vi "SR400 Control.vi"(0 "VISA Port In":refnum<visa-resource-name>="GPIB0::23::INSTR", 11 "error in":errorcluster) -> (4 "VISA Port Out":refnum<visa-resource-name>="SR400", 15 "error out":errorcluster)   [LabVIEW 2019]
doc: "Ce VI sert de centrale de contrôle pour le compteur de photon SR400. Il permet à l'usager de régler les différnet paramètres de comptage, de porte et de discriminateur."
uses:
  <vilib>/Utility/error.llb/DialogType.ctl
panel:
  in  "ReadPar":bool
  in  "Test":bool
  in  "BGatePar":T1={"Mode"=0, "Durée"=0.9992, "Délais"=0.9992, "Incrément"=0.9992} caption="Paramètres de la porte d'acquisition «B»" {"Incrément" min=0.0 max=0.9992 step=1e-09 format="%#_4g"; "Délais" min=0.0 max=0.9992 step=1e-09 format="%#_4g"; "Durée" min=5e-09 max=0.9992 step=1e-09 format="%#_4g"; "Mode" items=["CW", "Fixed", "Scan"]}
  in  "AGatePar":T1={"Mode"=0, "Durée"=0.9992, "Délais"=0.9992, "Incrément"=0.9992} caption="Paramètres de la porte d'acquisition «A»" {"Incrément" min=0.0 max=0.9992 step=1e-09 format="%#_4g"; "Délais" min=0.0 max=0.9992 step=1e-09 format="%#_4g"; "Durée" min=5e-09 max=0.9992 step=1e-09 format="%#_4g"; "Mode" items=["CW", "Fixed", "Scan"]}
  in  "Discriminateur T":T2 {"Incrément (V)" min=-0.02 max=0.02 step=0.0002; "Niveau (V)" min=-0.3 max=0.3 step=0.0002; "Front A" items=["Montant", "Descendant"]; "Mode" items=["Fixe", "Scan"]}
  in  "Discriminateur B":T2 {"Incrément (V)" min=-0.02 max=0.02 step=0.0002; "Niveau (V)" min=-0.3 max=0.3 step=0.0002; "Front A" items=["Montant", "Descendant"]; "Mode" items=["Fixe", "Scan"]}
  in  "Discriminateur A":T2 {"Incrément (V)" min=-0.02 max=0.02 step=0.0002; "Niveau (V)" min=-0.3 max=0.3 step=0.0002; "Front A" items=["Montant", "Descendant"]; "Mode" items=["Fixe", "Scan"]}
  in  "Counter T Preset (s)":dbl=0.001 min=1e-07 max=90000.0 step=1e-07 format="%#.7g"
  in  "Dwell time":dbl=6.0 caption="\"Dwell Time\" (s)" min=0.002 max=6.0 step=0.001
  in  "Mode":u16(ring) items=["A,B for T Preset", "A-B for T Preset", "A+B for T Preset", "A for B preset"]
  in  "Nb de période":i32=1 min=1 max=2000 step=1
  in  "Counter B Preset (s)":dbl=0.001 min=1e-07 max=90000.0 step=1e-07 format="%#.7g"
  in  "T Source":u16(ring) caption="Source «T»" items=["10 MHz"=0, "Input 2"=2, "Trig"=3]
  in  "B Source":u16(ring)=2 caption="Source «B»" items=["Input 1"=1, "Input 2"=2]
  in  "A Source":u16(ring)=1 caption="Source «A»" items=["Input 1"=1, "10 MHz"=0]
  in  "Quit":bool
  # "Panneaux de contrôle du Compteur de Photon SR400"
  # "Porte D'acquisition «Gate»"
  # "Source de comptage"
  # "Paramètres de comptage"
  # "Discriminateur"
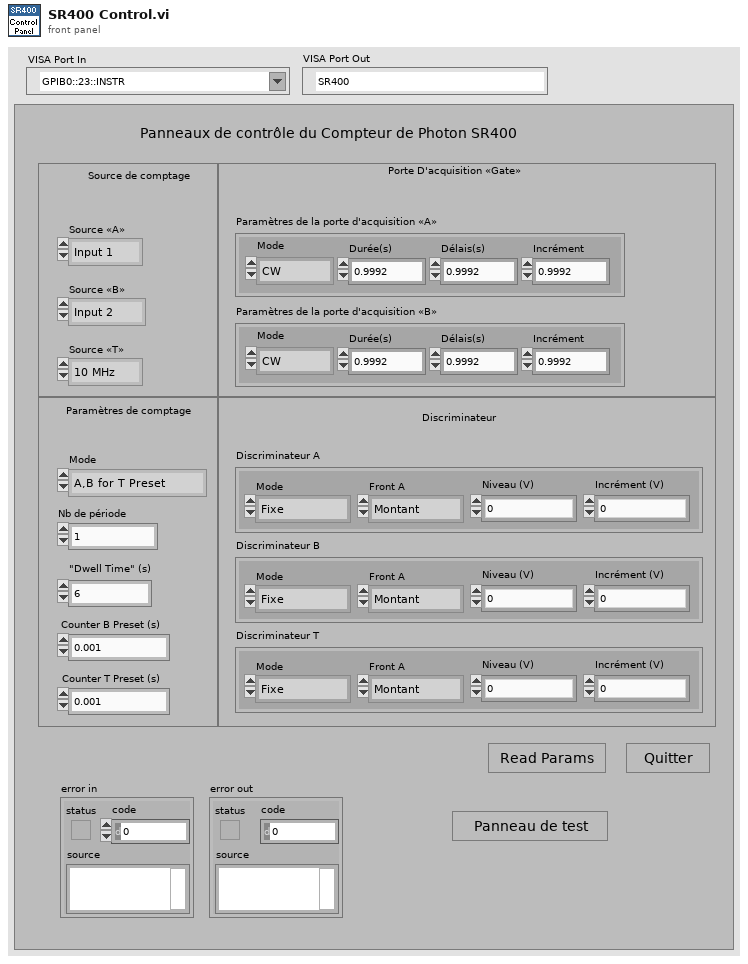
[diagram p1: front panel]
types:
  T1 = cluster{"Mode":u16, "Durée":dbl, "Délais":dbl, "Incrément":dbl}
  T2 = cluster{"Mode":u16, "Front A":u16, "Niveau (V)":dbl, "Incrément (V)":dbl}
  T3 = enum16{"All", "Mode", "T Preset", "B Preset", "Dwell", "NbPeriod", "Counter"}
  T4 = typedef "DialogType.ctl" = u16
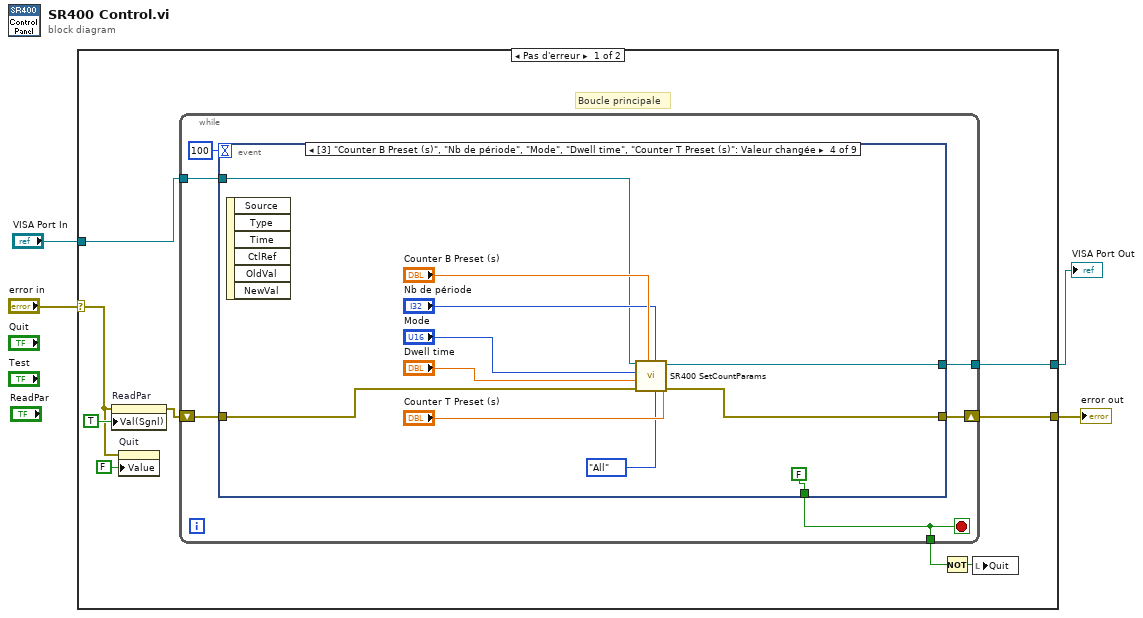
[diagram p0: block diagram]
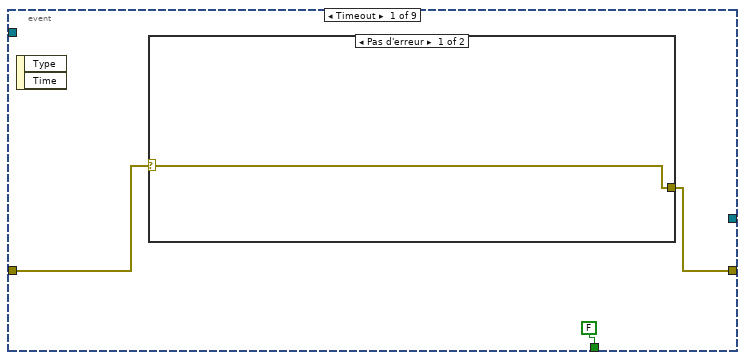
[diagram p2: hidden frame]
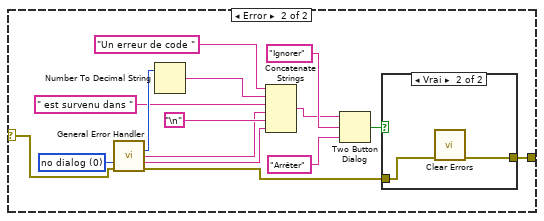
[diagram p3: hidden frame]
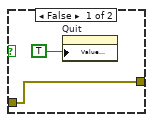
[diagram p4: hidden frame]
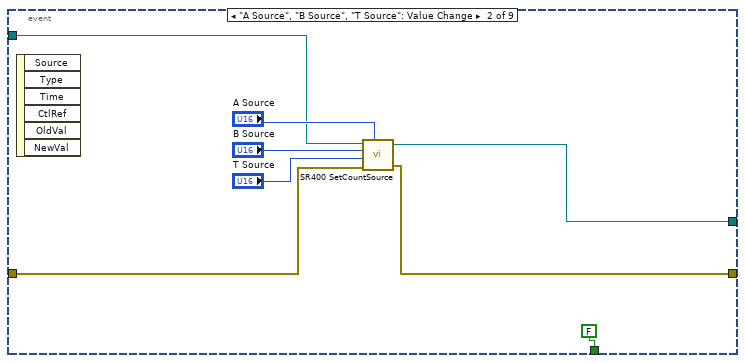
[diagram p5: hidden frame]
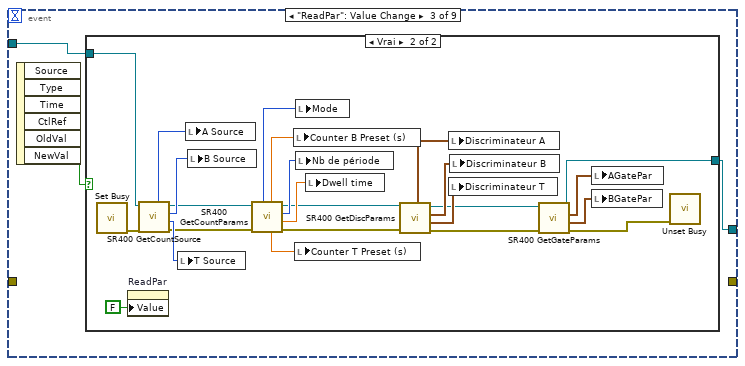
[diagram p6: hidden frame]
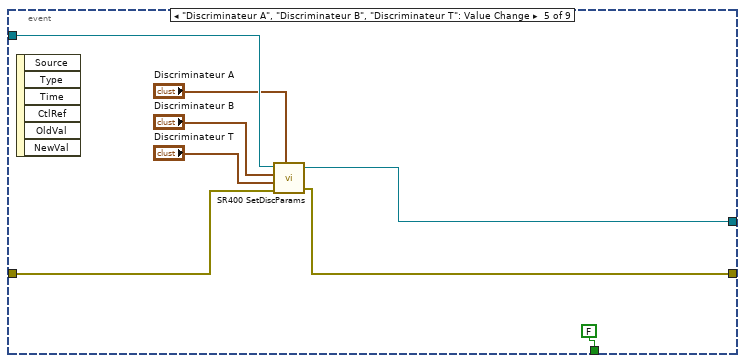
[diagram p8: hidden frame]
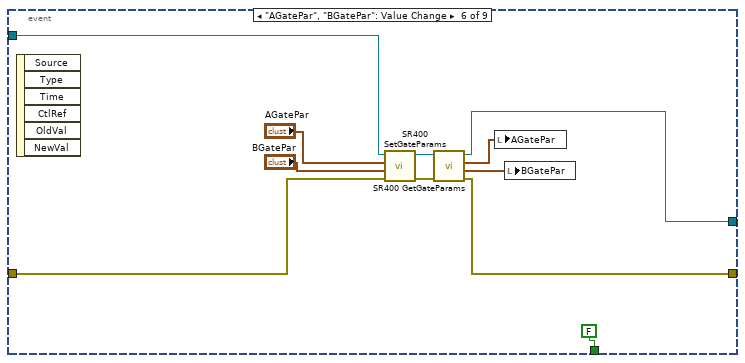
[diagram p9: hidden frame]
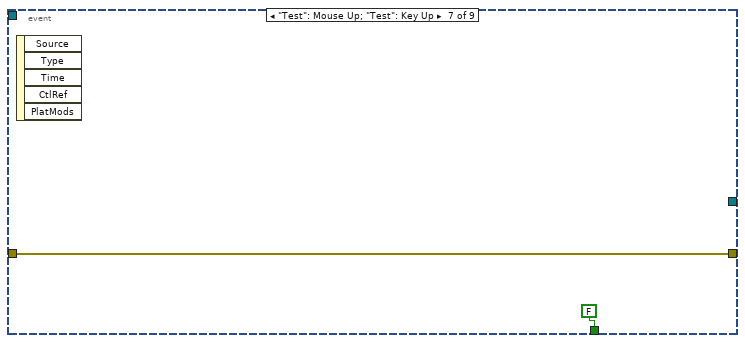
[diagram p10: hidden frame]
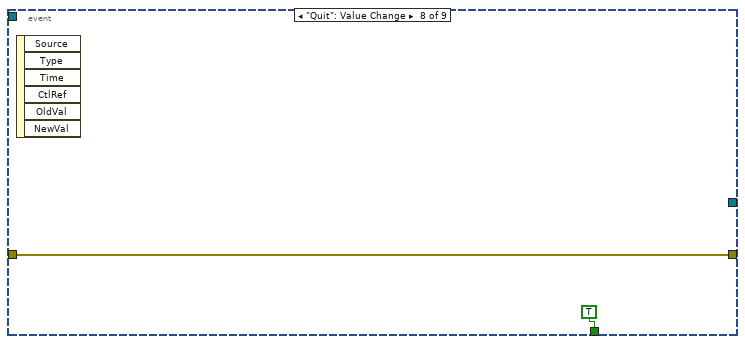
[diagram p11: hidden frame]
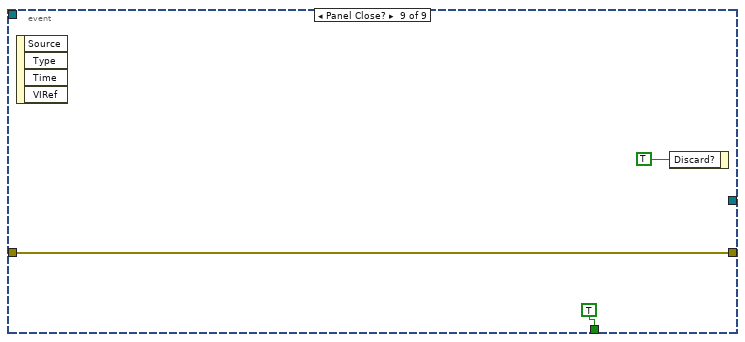
[diagram p12: hidden frame]
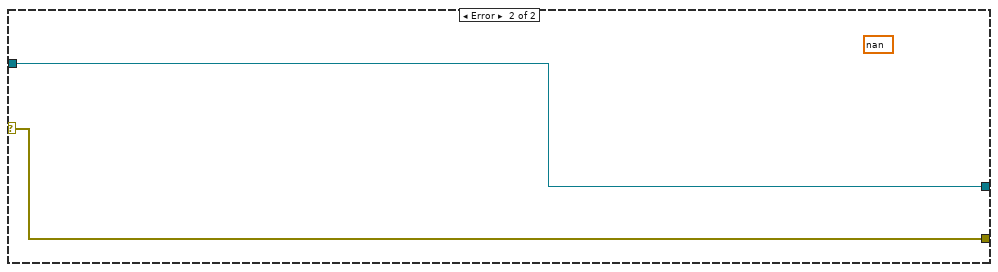
[diagram p13: hidden frame]
diagram:
  n1 = case shown="Pas d'erreur" "error in" {
    selector: "error in" -> [w5 w117]
    tunnel: [w13 w117] -> w3
    tunnel: "VISA Port In" -> [w7 w116]
    tunnel: [w12 w116] -> w1
    frame No Error {
      # "Boucle principale"
      n2 = property on="ReadPar" class="Bool (strict)"(error in=w5, "Val(Sgnl)"=TRUE ("Value (Signaling)")) -> (error out=w9:errorcluster)  [unwired: 1 in, 1 out]
      n3 = property on="Quit" class="Bool (strict)"(error in=w5, "Value"=FALSE ("Quit")) -> ()  [unwired: 1 in, 2 out]
      n4 = while {
        shift-right: [w17] -> w13
        shift-left: w9 -> [w18]
        tunnel: [w16] -> w11
        tunnel: w7 -> [w15]
        tunnel: [w14] -> w12
        stop <- w16 stop-if-true
        n5 = event shown="[3] \"Counter B Preset (s)\", \"Nb de période\", \"Mode\", \"Dwell time\", \"Counter T Preset (s)\": Valeur changée" {
          selector: _ -> [_ _ _ _ _ _ _ _ _]
          dyn-events: _ -> [_ _ _ _ _ _ _ _ _]
          timeout: 100 -> [_ _ _ _ _ _ _ _ _]
          tunnel: w18 -> [w20 w50 _ w89 w97 w108 w109 w111 w113]
          tunnel: [w21 w49 _ w88 w96 w106 w109 w111 w113] -> w17
          tunnel: [FALSE ("status") FALSE ("status") _ FALSE ("status") FALSE ("status") FALSE ("status") FALSE ("status") TRUE ("status") TRUE ("status")] -> w16
          tunnel: w15 -> [_ w44 w53 w81 w92 w101 _ _ _]
          tunnel: [_ w43 w52 w80 w90 w103 _ _ _] -> w14
          event Timeout {
            n6 = event-data() -> ()  [unwired: 1 in, 2 out]
            n7 = case shown="Pas d'erreur" w20 {
              selector: w20 -> [w23 w24]
              tunnel: [w23 w25] -> w21
              frame No Error {
              }
              frame Error {
                w35 = T4 0 items=["no dialog", "OK message", "continue or stop message", "OK message + warnings", "continue/stop + warnings"] ("type of dialog (OK msg:1)")
                n8 = call <vilib>:"General Error Handler.vi"("type of dialog (OK msg:1)"=w35, "error in (no error)"=w24) -> ("code out"=w31:i32, "source out"=w30:string, "message"=w28:string, "error out"=w26:errorcluster)  [unwired: 9 in, 1 out]
                n9 = Number To Decimal String(number=w31) -> (decimal integer string=w32:string)  [unwired: 1 in]
                n10 = Concatenate Strings("Un erreur de code " ("string"), w32, " est survenu dans " ("string"), w30, "\n", w28) -> (w27:string)
                n11 = Two Button Dialog(message=w27, 1:"Arrêter" ("F button name (\"Cancel\")"), 2:"Ignorer" ("T button name (\"OK\")")) -> (T button?=w38:bool)
                n12 = case shown="Vrai" w38 {
                  tunnel: w26 -> [w40 w42]
                  tunnel: [w40 w41] -> w25
                  frame False {
                    n13 = property on="Quit" class="Bool (strict)"("Value (Signaling)"=TRUE) -> ()  [unwired: 2 in, 2 out]
                  }
                  frame True {
                    n14 = call <vilib>:"Clear Errors.vi"("error in (no error)"=w42) -> ("error out"=w41:errorcluster)  [unwired: 5 in, 1 out]
                  }
                }
              }
            }
          }
          event "A Source", "B Source", "T Source": Value Change {
            n15 = event-data() -> ()  [unwired: 1 in, 6 out]
            n16 = call <userlib>:"SR400 SetCountSource.vi"("error in (no error)"=w50, "T Source"="T Source", "A Source"="A Source", "B Source"="B Source", "VISA Port In"=w44) -> ("error out"=w49:errorcluster, "VISA Port Out"=w43:refnum<visa-resource-name>)  [unwired: 4 in]
          }
          event "ReadPar": Value Change {
            n17 = event-data() -> ("NewVal"=w51:bool)  [unwired: 1 in, 5 out]
            n18 = case shown="Vrai" w51 {
              tunnel: w53 -> [w54 w58]
              tunnel: [w54 w57] -> w52
              frame False {
              }
              frame True {
                n19 = call <vilib>:"Set Busy.vi"() -> ("error out"=w69:errorcluster)  [unwired: 10 in, 1 out]
                n20 = property on="ReadPar" class="Bool (strict)"("Value"=FALSE ("ReadPar")) -> ()  [unwired: 2 in, 2 out]
                n21 = call <userlib>:"SR400 GetCountSource.vi"("error in (no error)"=w69, "VISA Port In"=w58) -> ("error out"=w77:errorcluster, "T Source"=w78:u16, "B Source"=w67:u16, "VISA Port Out"=w66:refnum<visa-resource-name>, "A Source"=w68:u16)  [unwired: 4 in]
                n22 = local write "T Source"(w78) -> ()
                n23 = local write "A Source"(w68) -> ()
                n24 = local write "B Source"(w67) -> ()
                n25 = call <userlib>:"SR400 GetCountParams.vi"("error in (no error)"=w77, "VISA Port In"=w66) -> ("error out"=w74:errorcluster, "Dwell time"=w76:dbl, "Nb de période"=w75:i32, "VISA Port Out"=w62:refnum<visa-resource-name>, "CounterPresT"=w64:dbl, "CounterPresB"=w65:dbl, "Mode"=w63:u16)  [unwired: 3 in]
                n26 = local write "Counter B Preset (s)"(w65) -> ()
                n27 = local write "Counter T Preset (s)"(w64) -> ()
                n28 = local write "Mode"(w63) -> ()
                n29 = local write "Nb de période"(w75) -> ()
                n30 = local write "Dwell time"(w76) -> ()
                n31 = call <userlib>:"SR400 GetDiscParams.vi"("error in (no error)"=w74, "VISA Port In"=w62) -> ("error out"=w70:errorcluster, "Discriminateur T"=w71:T2, "Discriminateur B"=w72:T2, "VISA Port Out"=w59:refnum<visa-resource-name>, "Discriminateur A"=w73:T2)  [unwired: 4 in]
                n32 = local write "Discriminateur A"(w73) -> ()
                n33 = local write "Discriminateur T"(w71) -> ()
                n34 = local write "Discriminateur B"(w72) -> ()
                n35 = call <userlib>:"SR400 GetGateParams.vi"("error in (no error)"=w70, "VISA Port In"=w59) -> ("error out"=w55:errorcluster, "BGatePar"=w61:T1, "AGatePar"=w60:T1, "VISA Port Out"=w57:refnum<visa-resource-name>)  [unwired: 6 in]
                n36 = local write "AGatePar"(w60) -> ()
                n37 = local write "BGatePar"(w61) -> ()
                n38 = call <vilib>:"Unset Busy.vi"("error in (no error)"=w55) -> ()  [unwired: 10 in, 1 out]
              }
            }
          }
          event "Counter B Preset (s)", "Nb de période", "Mode", "Dwell time", "Counter T Preset (s)": Value Change {
            n39 = event-data() -> ()  [unwired: 1 in, 6 out]
            n40 = call <userlib>:"SR400 SetCountParams.vi"("Counter T Preset (s)"="Counter T Preset (s)", "Operation"=T3."All", "Nb de période"="Nb de période", "Counter B Preset (s)"="Counter B Preset (s)", "error in (no error)"=w89, "Dwell time"="Dwell time", "Mode"="Mode", "VISA Port In"=w81) -> ("error out"=w88:errorcluster, "VISA Port Out"=w80:refnum<visa-resource-name>)  [unwired: 2 in]
          }
          event "Discriminateur A", "Discriminateur B", "Discriminateur T": Value Change {
            n41 = event-data() -> ()  [unwired: 1 in, 6 out]
            n42 = call <userlib>:"SR400 SetDiscParams.vi"("error in (no error)"=w97, "Discriminateur T"="Discriminateur T", "Discriminateur A"="Discriminateur A", "Discriminateur B"="Discriminateur B", "VISA Port In"=w92) -> ("error out"=w96:errorcluster, "VISA Port Out"=w90:refnum<visa-resource-name>)  [unwired: 4 in]
          }
          event "AGatePar", "BGatePar": Value Change {
            n43 = event-data() -> ()  [unwired: 1 in, 6 out]
            n44 = call <userlib>:"SR400 SetGateParams.vi"("error in (no error)"=w108, "BGatePar"="BGatePar", "AGatePar"="AGatePar", "VISA Port In"=w101) -> ("error out"=w107:errorcluster, "VISA Port Out"=w102:refnum<visa-resource-name>)  [unwired: 4 in]
            n45 = call <userlib>:"SR400 GetGateParams.vi"("error in (no error)"=w107, "VISA Port In"=w102) -> ("error out"=w106:errorcluster, "BGatePar"=w105:T1, "AGatePar"=w98:T1, "VISA Port Out"=w103:refnum<visa-resource-name>)  [unwired: 6 in]
            n46 = local write "AGatePar"(w98) -> ()
            n47 = local write "BGatePar"(w105) -> ()
          }
          event "Test": Mouse Up; "Test": Key Up {
            n48 = event-data() -> ()  [unwired: 1 in, 5 out]
          }
          event "Quit": Value Change {
            n49 = event-data() -> ()  [unwired: 1 in, 6 out]
          }
          event Panel Close? {
            n50 = event-data() -> ()  [unwired: 1 in, 4 out]
            n51 = event-data("Discard?"=TRUE) -> ()  [unwired: 1 in, 1 out]
          }
        }
      }
      n52 = Not(x=w11) -> (.not. x?=w10:bool)
      n53 = local write "Quit"(w10) -> ()
    }
    frame Error {
      (unwired) nan ("Wavelenght")
    }
  }
  "error out" <- w3
  "VISA Port Out" <- w1
